vi "HEWH RLT Label Parse.vi"(8 "Error In":errorcluster, 11 "Station A":T1) -> (0 "Error Out":errorcluster, 2 "Agilent Channel List":string[][](array[string]), 3 "MW100 Channel List":string[][](array[string]), 4 "Agilent Labels":string[](array[string]), 6 "MW100 Labels":string[](array[string]))   [LabVIEW 2020]
uses:
  Type Definitions/HEWH RLT Stations.ctl
  Type Definitions/HEWH Label Channel.ctl
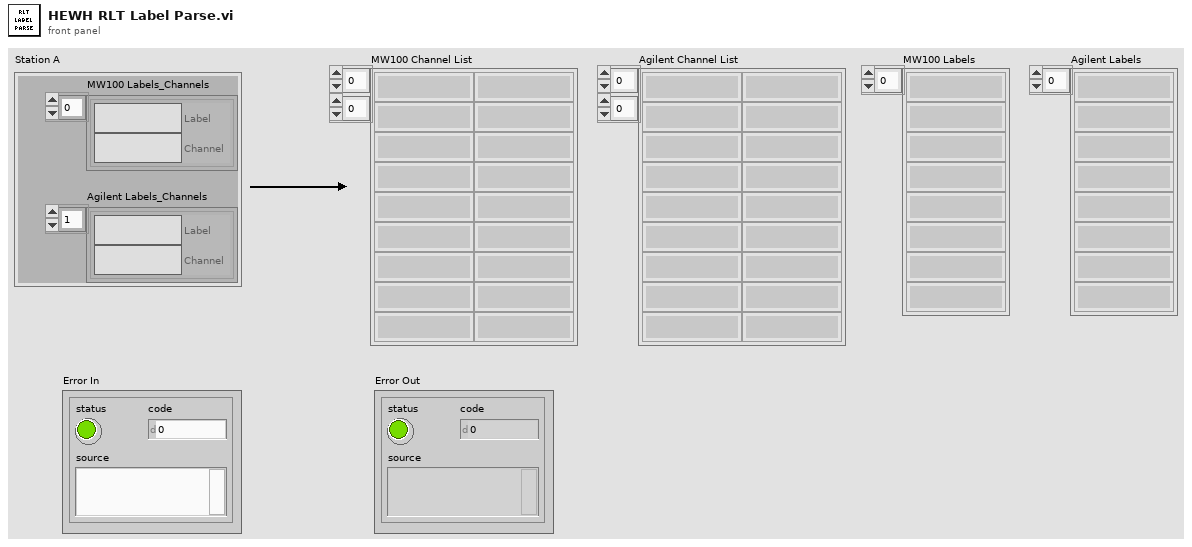
[diagram p1: front panel]
types:
  T1 = typedef "HEWH RLT Stations.ctl" = cluster{"MW100 Labels_Channels":T2[], "Agilent Labels_Channels":T2[]}
  T2 = typedef "HEWH Label Channel.ctl" = cluster{"Label":string, "Channel":string}
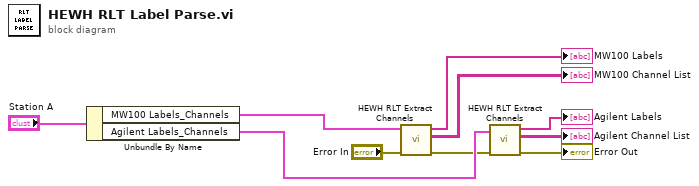
[diagram p0: block diagram]
diagram:
  n1 = Unbundle By Name("Station A") -> ("MW100 Labels_Channels"=w6:T2[], "Agilent Labels_Channels"=w9:T2[])
  n2 = call "HEWH RLT Extract Channels.vi"("Error In"="Error In", "Agilent Labels_Channels"=w6) -> ("Error Out"=w5:errorcluster, "Channels"=→"MW100 Channel List":string[][], "Lables"=→"MW100 Labels":string[])  [unwired: 7 in]
  n3 = call "HEWH RLT Extract Channels.vi"("Error In"=w5, "Agilent Labels_Channels"=w9) -> ("Error Out"=→"Error Out":errorcluster, "Channels"=→"Agilent Channel List":string[][], "Lables"=→"Agilent Labels":string[])  [unwired: 7 in]
